vi "INI-FP.vi"(6 "Mode":enum16{"Read", "Write"}(ring)=enum."Write", 7 "prompt":string="Please select or create config file", 8 "section":string, 9 "Controls[]":refnum<vi>[](array[refnum]), 10 "VIreference":refnum<vi>, 11 "INIfilepathIn":path) -> (0 "error out":errorcluster, 3 "INIfilepathOut":path)   [LabVIEW 2021]
uses:
  varDescriptor.ctl
  <vilib>/Utility/Data Type/Type Definitions/Data Type.ctl
  <vilib>/Utility/config.llb/NI_LVConfig.lvlib
  <vilib>/Utility/Data Type/NI_Data Type.lvlib
panel:
  out "nControls":i32
  out "varDesciptions":T1[](array[typedef])
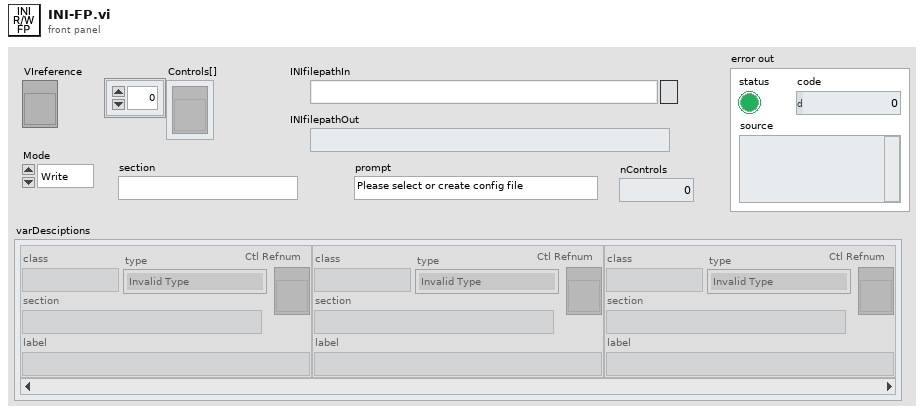
[diagram p1: front panel]
types:
  T1 = typedef "varDescriptor.ctl" = cluster{"class":string, "type":T2, "section":string, "label":string, "Ctl Refnum":refnum<vi>}
  T2 = typedef "NI_Data Type.lvlib/Data Type.ctl" = enum8{"Invalid Type", "Void", "I8", "I16", "I32", "I64", "U8", "U16", "U32", "U64", "Single Float", "Double Float", "Extended Float", "Single Complex", "Double Complex", "Extended Complex", "Enum U8", "Enum U16", "Enum U32", "Enum U64", "Single Float With Unit", "Double Float With Unit", "Extended Float With Unit", "Single Complex with Unit", "Double Complex with Unit", "Extended Complex with Unit", "Boolean", "String", "Path", "Picture", "Tag", "Array", "Cluster", "Variant", "LV Variant", "Waveform", "Timestamp", "Digital Waveform", "Digital Data", "ExpressData", "Refnum", "External Data", "VI", "Poly VI", "LabVIEW Class Instance", "Fixed Point", "Set Collection", "Map Collection"}
  T3 = typedef "NI_LVConfig.lvlib/Config Data RefNum.ctl" = refnum<k1>
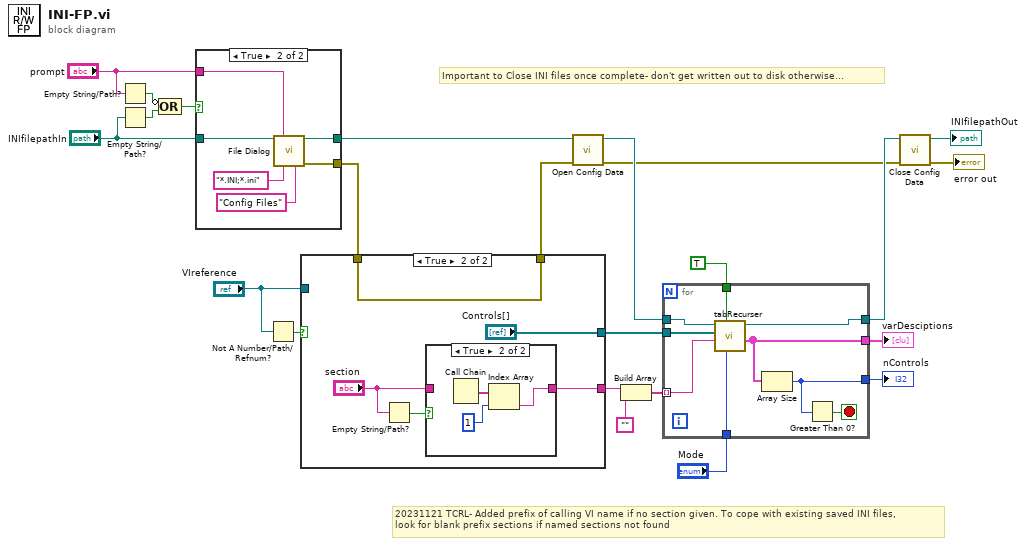
[diagram p0: block diagram]
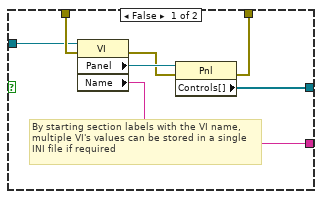
[diagram p2: hidden frame]
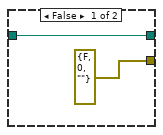
[diagram p4: hidden frame]
diagram:
  # "20231121 TCRL- Added prefix of calling VI name if no section given. To cope with existing saved INI files,\nlook for blank prefix sections if named sections not found"
  # "Important to Close INI files once complete- don't get written out to disk otherwise..."
  n1 = Empty String/Path?(string/path="prompt") -> (empty?=w20:bool)
  n2 = Empty String/Path?(string/path="INIfilepathIn") -> (empty?=w21:bool)
  n3 = Compound Arithmetic op=OR(invert w20, w21) -> (w22:bool)
  n4 = case shown="True" w22 {
    tunnel: "INIfilepathIn" -> [w25 w28]
    tunnel: [w25 w31] -> w16
    tunnel: "prompt" -> [_ w27]
    tunnel: [errorcluster {"status"=FALSE, "code"=0, "source"=""} ("error out") w26] -> w11
    frame False {
    }
    frame True {
      n5 = call "File Dialog"("start path"=w28, "prompt"=w27, "pattern (all files)"="*.INI;*.ini", "pattern label"="Config Files") -> ("selected path"=w31:path, "error out"=w26:errorcluster)  [unwired: 8 in, 2 out]
    }
  }
  n6 = Not A Number/Path/Refnum?(number/path/refnum="VIreference") -> (NaN/Path/Refnum?=w4:bool)
  n7 = case shown="True" w4 {
    tunnel: [w37 w40] -> w23
    tunnel: [w36 "Controls[]"] -> w17
    tunnel: w11 -> [w34 w43]
    tunnel: [w33 w43] -> w10
    tunnel: "VIreference" -> [w32 _]
    frame False {
      # "By starting section labels with the VI name, multiple VI's values can be stored in a single INI file if required"
      n8 = property class="VI"(reference=w32, error in=w34) -> (error out=w35:errorcluster, "Panel"=w38:refnum<vi>, "Name"=w37:string)  [unwired: 1 out]
      n9 = property on="Property Node" class="Pnl"(reference=w38, error in=w35) -> (error out=w33:errorcluster, "Controls[]"=w36:refnum<vi>[])  [unwired: 1 out]
    }
    frame True {
      n10 = Empty String/Path?(string/path="section") -> (empty?=w41:bool)
      n11 = case shown="True" w41 {
        tunnel: [w44 w47] -> w40
        tunnel: "section" -> [w44 _]
        frame False {
        }
        frame True {
          n12 = Call Chain() -> (call chain=w46:string[])
          n13 = Index Array(array=w46, index=1) -> (element=w47:string)
        }
      }
    }
  }
  n14 = call <vilib>:"Open Config Data.vi"("error in (no error)"=w10, "configuration file path"=w16) -> ("error out"=w12:errorcluster, "refnum"=w15:T3)  [unwired: 7 in, 1 out]
  n15 = Build Array(w23, "") -> (w3:string[])
  n16 = for {
    tunnel: w17 -> [w56]
    tunnel: "Mode" -> [w53]
    tunnel: [w52] -> w9
    tunnel: [w49] -> w8
    tunnel: w3 -> [w51] mode=indexing
    tunnel: w15 -> [w55]
    tunnel: [w54] -> w14
    tunnel: TRUE ("controlsOnly") -> [w48]
    stop <- w50 stop-if-true
    n17 = call "tabRecurser.vi"("Mode"=w53, "controlsOnly"=w48, "SectionNameIn"=w51, "controlsIn[]"=w56, "INIrefnumIn"=w55) -> ("varDescriptions"=w52:T1[], "INIrefnumOut"=w54:T3)  [unwired: 5 in]
    n18 = Array Size(array=w52) -> (size(s)=w49:i32)
    n19 = Greater Than 0?(x=w49) -> (x > 0?=w50:bool)
  }
  "varDesciptions" <- w9
  "nControls" <- w8
  n20 = call <vilib>:"Close Config Data.vi"("error in (no error)"=w12, "refnum"=w14) -> ("error out"=→"error out":errorcluster, "file path"=→"INIfilepathOut":path)  [unwired: 8 in]
